vi "BK Precision 1696.vi"() -> ()   [LabVIEW 2020]
uses:
  SubVIs/BK_Precision1696_TypeDefinitions.llb/BK_1696_Output_On_OFF.ctl
  SubVIs/BK_Precision1696_TypeDefinitions.llb/BK_Precision1696_Steps.ctl
  LabVIEW 2020 Toolkits/toolkits_lv2020_32bit/Synchronization.llb/SynchRefs_SetGet.ctl
  LabVIEW 2020 Toolkits/VI Server Toolkit/VI Server Libraries/VI Server_Set Controls.llb/Set STR Control.vi
  LabVIEW 2020 Toolkits/VI Server Toolkit/VI Server Toolkit LV2013.lvlib
panel:
  out "InstrumentGood":bool caption="Instrument Good"
  out "InterfaceError":bool caption="Interface Error"
  out "CommandStatus":bool caption="Command Status"
  out "System.Message":string caption="System Message"
  in  "Help":bool
  in  "FP.Hide":bool caption="FrontPanel.Hide"
  in  "EXIT":bool
  in  "error in":errorcluster
  in  "Tab.Main":T1(tab)
  out "Indicator.CV":bool
  in  "Indicator.OVP.Set":dbl caption="Indicator.Current.Measured" format="%0.1f"
  in  "Indicator.Current.Set":dbl caption="Indicator.Current.Measured" format="%0.2f"
  in  "Indicator.Voltage.Set":dbl=0.1 caption="Indicator.Voltage.Measured" min=0.1 max=20.0 format="%0.1f "
  out "Indicator.Output.Enabled":T2
  in  "Indicator.Current.Measured":dbl format="%0.3f"
  in  "Indicator.Voltage.Measured":dbl format="%0.2f "
  in  "Indicator.Power.Measured":dbl format="%0.3f"
  in  "OVP.Level":dbl caption="OVP.Level.DUP" min=0.0 max=20.0 format="%0.1f V"
  in  "OVP.Level.DUP":dbl(knob) caption="Volts" min=0.0 max=20.0 scale=0.0..20.0
  in  "Output.Amps":dbl caption="Output.Amps.DUP" min=0.0 max=80.0 format="%0.3f A"
  in  "Output.Amps.DUP":dbl(knob) caption="Current Limit (Amp)" min=0.0 max=10.0 scale=0.0..10.0
  in  "Output.Volts":dbl=1.0 caption="Output.Volts.DUP" min=1.0 max=20.0 format="%0.1f V"
  in  "Output.Volts.DUP":dbl(knob)=1.0 caption="Volts" min=1.0 max=20.0 scale=1.0..20.0
  in  "Output.Enable":bool
  out "List.File.LoadedStep":string caption="Loaded Step"
  in  "List.File.#Cycles":u16 caption="# of Cycles" max=256 format="%03d"
  in  "List.File.Description":string caption="File Description"
  in  "List.File.Open":bool
  in  "List.File.RUN":bool
  in  "List.File.Load":bool
  in  "List.File.Save":bool
  in  "List.File":u16=1 caption="List File" min=1 max=100
  in  "Step.Parameters":T3 caption="Program Parameters" {"Seconds" max=59; "Minutes" max=99; "Step.Current" format="%0.2f A"; "Step.Voltage" format="%0.1f V"}
  in  "List.File.RUN.DUP":bool caption="List.File.RUN"
  out "Program.Progress":u8(slide) caption="Program Progress" scale=0.0..100.0
  out "Graph.TimeBetweenPoints":i32 caption="Time Between Points" format="%.0f msec"
  in  "Graph.Enable":bool
  out "Sequence.Graph":cluster{i32[], dbl[]}[](graph)
  in  "Instrument.Address":u8 caption="Instrument Address" max=31 format="%03d"
  in  "Measurements.AutoUpdate.Disable":bool
  in  "Measurements.UpdateRate":u32=100 caption="Measurements Update Rate" min=100 max=100000 format="%.0f msec"
  in  "VISA.Command2.Write":bool
  in  "VISA.Command2":string caption="Command"
  in  "VISA.Command.Write":bool
  in  "VISA.Command":string caption="Command"
  out "VISA.InstrumentResponce":string caption="Instrument Responce"
  in  "VISA.ResourceName":refnum<visa-resource-name>="BK_PRECISION_9115" caption="VISA Rresource Name"
  in  "UDP.Test.String2.Send":bool
  in  "UDP.Test.String2":string caption="UDP: Test String 2"
  in  "UDP.Port.Receiver":u16=58433 caption="UDP: Port.Receiver"
  in  "UDP.Port.Read":u16=58432 caption="UDP: Port.Read"
  in  "UDP.LocalPort.Write":u16=58434 caption="UDP: Local Port.Write"
  in  "UDP.IP.Address":string="234.5.6.7" caption="UDP: IP Address"
  in  "UDP.Test.String1.Send":bool
  in  "UDP.Test.String1":string caption="UDP: Test String 1"
  in  "UDP.Responce.String.Monitor":bool
  out "UDP.Responce.String":string caption="UDP: Responce String"
  in  "VI.WindowsTitle":string caption="Windows Title"
  out "error out":errorcluster={"status"=TRUE, "code"=1055, "source"="Property Node in VI Server Toolkit LV2013.lvlib:VI server_Set Control Value from String Format.vi:5200001->DMM6500_UDP_ExecEng_Instruction_APPLY.vi->DMM6500_UDP_MAIN.vi->Keithley2100.vi"}
  # "V"
  # "[SETTINGS]"
  # "V"
  # "V-set"
  # "A"
  # "A"
  # "W"
  # "V"
  # "OVP"
  # "OUTPUT"
  # "OUTPUT"
  # "OVERVOLTAGE"
  # "Step #               Voltage                  Current               Minute      Seconds"
  # "RS232 -> 000\nRS485 ->0 01 to 031"
  # "Multicast IP addresses must be in the 224.0.0.0 to 239.255.255.255 range."
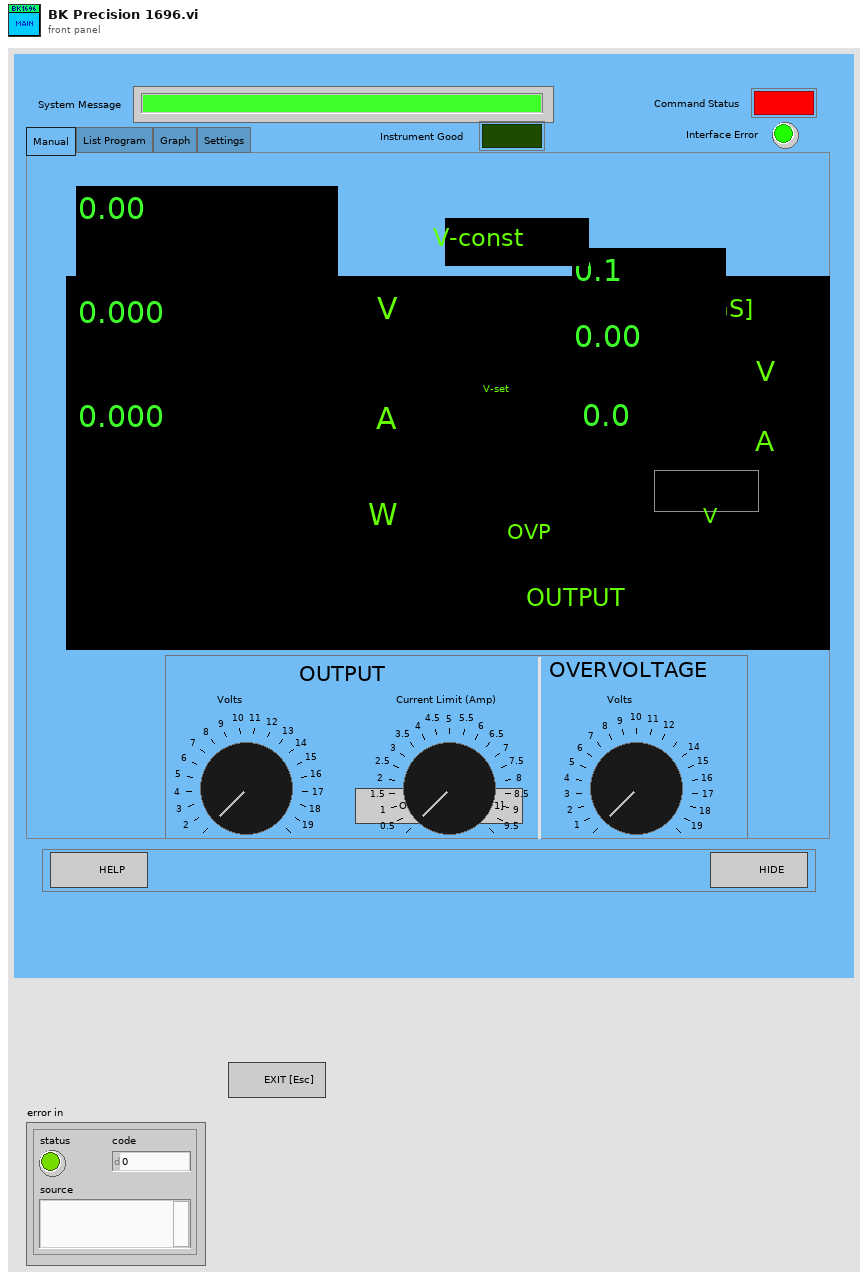
[diagram p1: front panel]
types:
  T1 = enum32{"Manual", "List Program", "Graph", "Settings"}
  T2 = typedef "BK_1696_Output_On_OFF.ctl" = bool
  T3 = typedef "BK_Precision1696_Steps.ctl" = cluster{"Step.Voltage":dbl, "Step.Current":dbl, "Minutes":u16, "Seconds":u16}[]
  T4 = typedef "VI Server_RefsCluster.ctl" = cluster{"Labels":string[], "Refs":refnum<vi>[], "VI Ref":refnum<vi>}
  T5 = typedef "SynchRefs_SetGet.ctl" = enum16{"Set", "Get"}
  T6 = cluster{"Step.Voltage":dbl, "Step.Current":dbl, "Step.Width":dbl, "Step.Slope":u8}[]
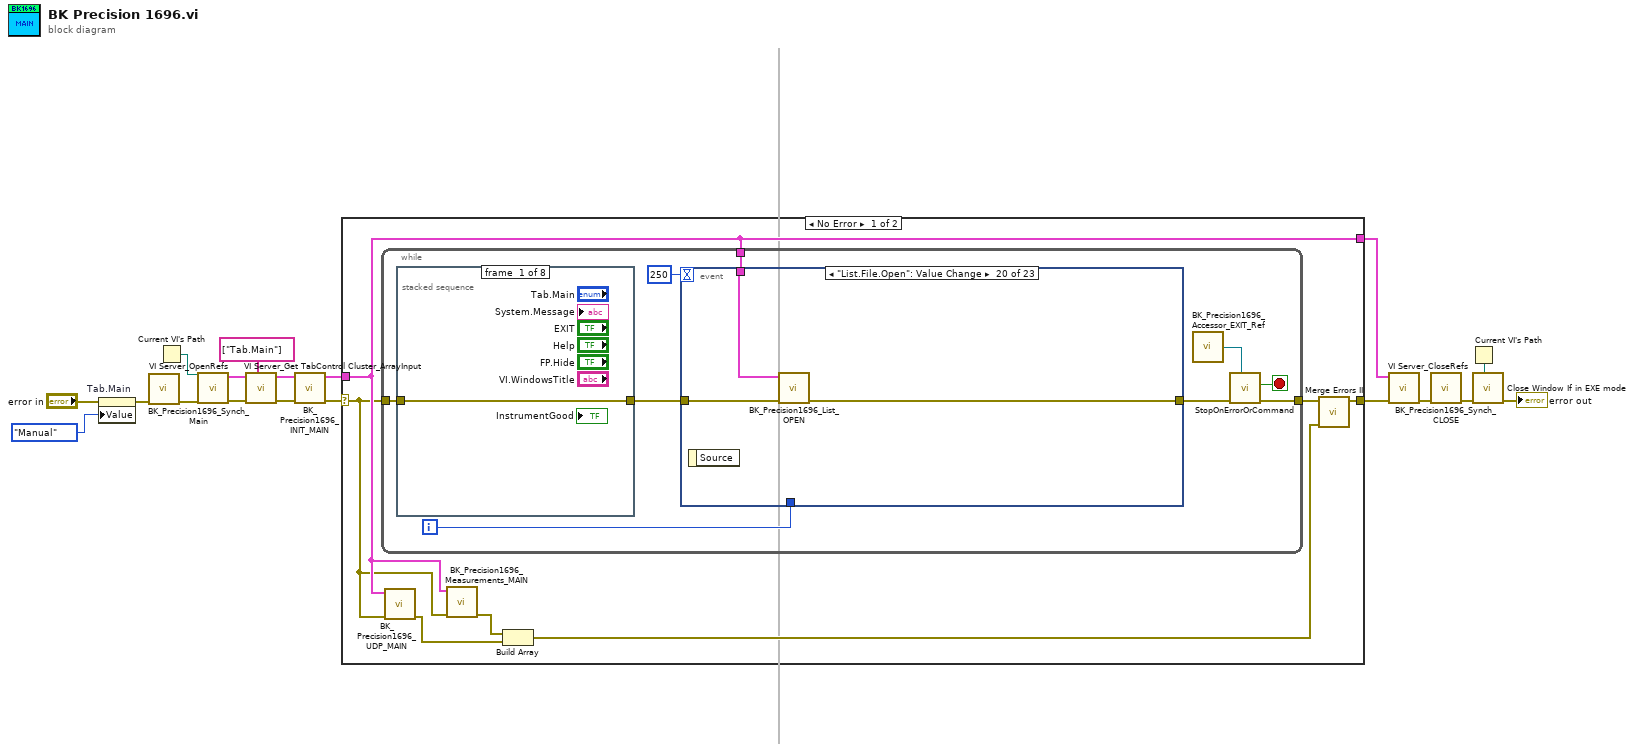
[diagram p0: block diagram]
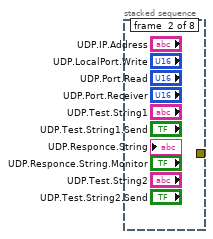
[diagram p2: hidden frame]
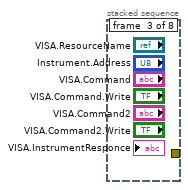
[diagram p3: hidden frame]
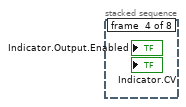
[diagram p4: hidden frame]
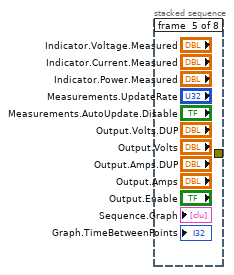
[diagram p5: hidden frame]
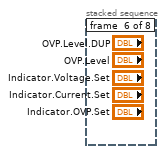
[diagram p6: hidden frame]
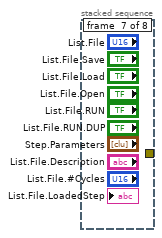
[diagram p7: hidden frame]
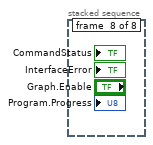
[diagram p8: hidden frame]
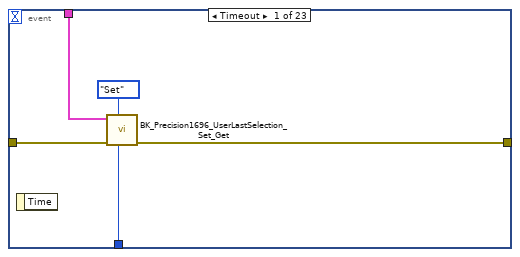
[diagram p9: hidden frame]
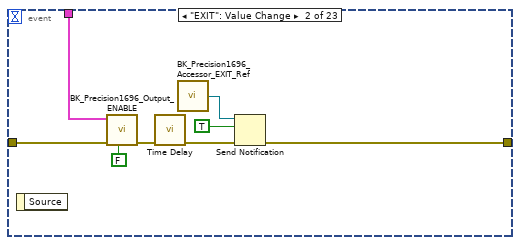
[diagram p10: hidden frame]
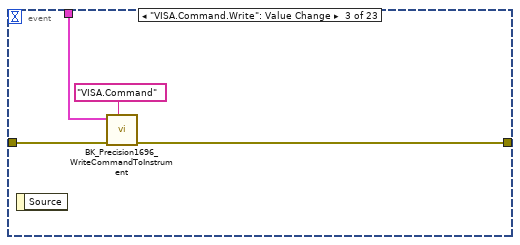
[diagram p11: hidden frame]
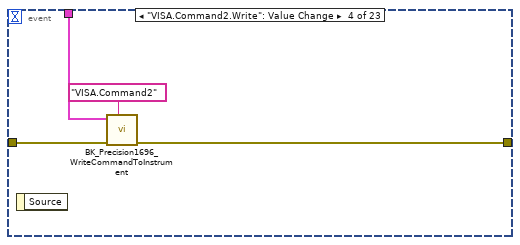
[diagram p12: hidden frame]
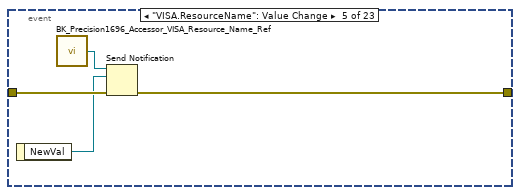
[diagram p13: hidden frame]
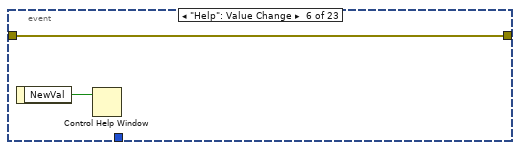
[diagram p14: hidden frame]
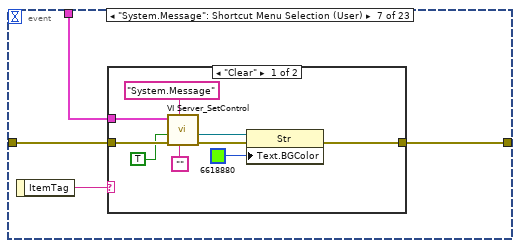
[diagram p15: hidden frame]
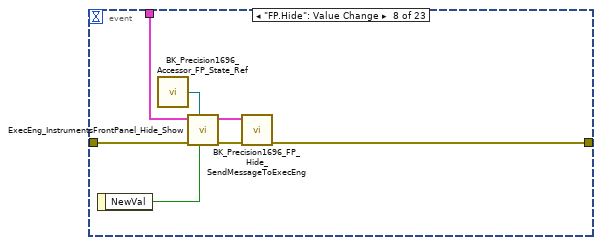
[diagram p17: hidden frame]
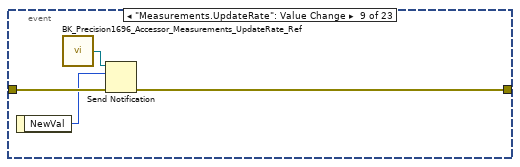
[diagram p18: hidden frame]
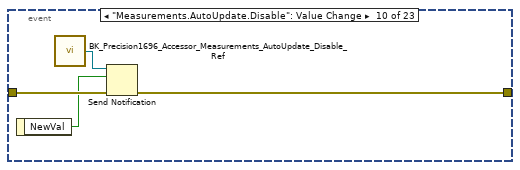
[diagram p19: hidden frame]
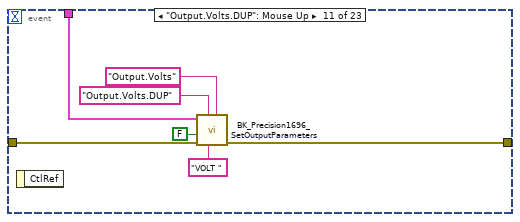
[diagram p20: hidden frame]
diagram:
  n1 = property on="Tab.Main" class="TabCtl (strict)"(error in="error in", "Value"=T1."Manual" ("Tab.Main")) -> (error out=w2:errorcluster)  [unwired: 1 in, 1 out]
  n2 = call "BK_Precision1696_Synch_Main.vi"("error in"=w2) -> ("error out"=w15:errorcluster)  [unwired: 10 in]
  n3 = Current VI's Path() -> (path=w17:path)
  n4 = call "VI Server_OpenRefs.vi"("error in"=w15, "VI Path"=w17) -> ("error out"=w14:errorcluster, "VI Server.RefsCluster"=w16:T4)  [unwired: 8 in]
  n5 = call "VI Server_Get TabControl Cluster_ArrayInput.vi"("TabControl Labels[]"=string[] ["Tab.Main"], "error in"=w14, "VI Server Cluster"=w16) -> ("error out"=w9:errorcluster, "VI Server Cluster.OUT"=w8:T4)  [unwired: 7 in]
  n6 = call "BK_Precision1696_INIT_MAIN.vi"("error in (no error)"=w9, "VI Server Cluster"=w8) -> ("error out"=w7:errorcluster, "VI Server Cluster DUP"=w5:T4)  [unwired: 8 in]
  n7 = case shown="No Error" w7 {
    selector: w7 -> [w22 w177]
    tunnel: [w24 w177] -> w6
    tunnel: w5 -> [w23 w176]
    tunnel: [w23 w176] -> w4
    frame No Error {
      n8 = while {
        tunnel: w22 -> [w34]
        tunnel: w23 -> [w31]
        tunnel: [w27] -> w25
        i -> [w30]
        stop <- w26 stop-if-true
        n9 = stacked-sequence {
          tunnel: w34 -> [w35 _ _ _ _ _ _ _]
          tunnel: [w35 _ _ _ _ _ _ _] -> w32
          frame #0 {
          }
          frame #1 {
          }
          frame #2 {
          }
          frame #3 {
          }
          frame #4 {
          }
          frame #5 {
          }
          frame #6 {
          }
          frame #7 {
          }
        }
        n10 = event shown="[19] \"List.File.Open\": Value Change" {
          selector: _ -> [_ _ _ _ _ _ _ _ _ _ _ _ _ _ _ _ _ _ _ _ _ _ _]
          dyn-events: _ -> [_ _ _ _ _ _ _ _ _ _ _ _ _ _ _ _ _ _ _ _ _ _ _]
          timeout: 250 -> [_ _ _ _ _ _ _ _ _ _ _ _ _ _ _ _ _ _ _ _ _ _ _]
          tunnel: w32 -> [w40 w44 w52 w56 w60 w61 w65 w83 w87 w91 w97 w104 w111 w118 w122 w129 w136 w151 w160 w163 w166 w171 w175]
          tunnel: w31 -> [w39 w45 w51 w55 _ _ w63 w81 _ _ w96 w103 w110 w117 w121 w128 w135 w152 w159 w162 w164 w170 _]
          tunnel: [w36 w47 w50 w54 w57 w61 w64 w78 w84 w89 w98 w105 w112 w119 w123 w130 w137 w142 w158 w161 w165 w169 w172] -> w28
          tunnel: w30 -> [w38 _ _ _ _ _ _ _ _ _ _ _ _ _ _ _ _ _ _ _ _ _ _]
          event Timeout {
            n11 = event-data() -> ()  [unwired: 1 in, 1 out]
            n12 = call "BK_Precision1696_UserLastSelection_Set_Get.vi"("LoopCounter"=w38, "SynchRefs.Set/Get"=SynchRefs_SetGet."Set", "error in"=w40, "VI Server.RefsCluster"=w39) -> ("error out"=w36:errorcluster)  [unwired: 6 in, 1 out]
          }
          event "EXIT": Value Change {
            n13 = event-data() -> ()  [unwired: 1 in, 1 out]
            n14 = call "BK_Precision1696_Output_ENABLE.vi"("Output.Enable"=FALSE, "error in (no error)"=w44, "VI Server Cluster"=w45) -> ("error out"=w41:errorcluster)  [unwired: 8 in]
            n15 = call "Time Delay"("error in (no error)"=w41) -> ("error out"=w42:errorcluster)  [unwired: 10 in]
            n16 = call "BK_Precision1696_Accessor_EXIT_Ref.vi"() -> ("EXIT"=w48:refnum<notifier>)  [unwired: 6 in]
            n17 = Send Notification(notification=TRUE, notifier=w48, error in (no error)=w42) -> (error out=w47:errorcluster)  [unwired: 1 out]
          }
          event "VISA.Command.Write": Value Change {
            n18 = event-data() -> ()  [unwired: 1 in, 1 out]
            n19 = call "BK_Precision1696_WriteCommandToInstrument.vi"("Control.Label"="VISA.Command", "error in (no error)"=w52, "VI Server Cluster"=w51) -> ("error out"=w50:errorcluster)  [unwired: 8 in]
          }
          event "VISA.Command2.Write": Value Change {
            n20 = event-data() -> ()  [unwired: 1 in, 1 out]
            n21 = call "BK_Precision1696_WriteCommandToInstrument.vi"("Control.Label"="VISA.Command2", "error in (no error)"=w56, "VI Server Cluster"=w55) -> ("error out"=w54:errorcluster)  [unwired: 8 in]
          }
          event "VISA.ResourceName": Value Change {
            n22 = event-data() -> ("NewVal"=w58:refnum<visa-resource-name>)  [unwired: 1 in]
            n23 = call "BK_Precision1696_Accessor_VISA_Resource_Name_Ref.vi"() -> ("VISA resource name"=w59:refnum<notifier>)  [unwired: 6 in]
            n24 = Send Notification(notification=w58, notifier=w59, error in (no error)=w60) -> (error out=w57:errorcluster)  [unwired: 1 out]
          }
          event "Help": Value Change {
            n25 = event-data() -> ("NewVal"=w62:bool)  [unwired: 1 in]
            n26 = Control Help Window(1:w62) -> ()  [unwired: 1 in]
          }
          event "System.Message": Shortcut Menu Selection (User) {
            n27 = event-data() -> ("ItemTag"=w66:string)  [unwired: 1 in]
            n28 = case shown="\"Clear\"" w66 {
              tunnel: w65 -> [w71 w76]
              tunnel: [w72 w76] -> w64
              tunnel: w63 -> [w69 _]
              frame "Clear" {
                n29 = call-poly "VI Server_SetControl.vi"("New Value"="", "Label"="System.Message", "error in"=w71, "Single Instance (T)"=TRUE ("SingleInstance"), "VI Server Cluster"=w69) -> ("error out"=w74:errorcluster, "Control Ref"=w75:refnum<vi>)  [unwired: 4 in, 1 out]
                n30 = property class="Str"(reference=w75, error in=w74, "Text.BGColor"=u32 6618880) -> (error out=w72:errorcluster)  [unwired: 1 out]
              }
              frame "", Default {
              }
            }
          }
          event "FP.Hide": Value Change {
            n31 = event-data() -> ("NewVal"=w82:bool)  [unwired: 1 in]
            n32 = call "BK_Precision1696_Accessor_FP_State_Ref.vi"() -> ("FP.State"=w80:refnum<notifier>)  [unwired: 6 in]
            n33 = call "ExecEng_InstrumentsFrontPanel_Hide_Show.vi"("FP.Hide/Show"=w82, "FP.State"=w80, "error in (no error)"=w83, "VI Server Cluster"=w81) -> ("error out"=w79:errorcluster, "VI Server Cluster DUP"=w77:T4)  [unwired: 6 in]
            n34 = call "BK_Precision1696_FP_Hide_SendMessageToExecEng.vi"("error in (no error)"=w79, "VI Server Cluster"=w77) -> ("error out"=w78:errorcluster)  [unwired: 9 in]
          }
          event "Measurements.UpdateRate": Value Change {
            n35 = event-data() -> ("NewVal"=w85:u32)  [unwired: 1 in]
            n36 = call "BK_Precision1696_Accessor_Measurements_UpdateRate_Ref.vi"() -> ("Measurements.UpdateRate"=w86:refnum<notifier>)  [unwired: 6 in]
            n37 = Send Notification(notification=w85, notifier=w86, error in (no error)=w87) -> (error out=w84:errorcluster)  [unwired: 1 out]
          }
          event "Measurements.AutoUpdate.Disable": Value Change {
            n38 = event-data() -> ("NewVal"=w90:bool)  [unwired: 1 in]
            n39 = call "BK_Precision1696_Accessor_Measurements_AutoUpdate_Disable_Ref.vi"() -> ("Measurements.AutoUpdate.Disable"=w88:refnum<notifier>)  [unwired: 6 in]
            n40 = Send Notification(notification=w90, notifier=w88, error in (no error)=w91) -> (error out=w89:errorcluster)  [unwired: 1 out]
          }
          event "Output.Volts.DUP": Mouse Up {
            n41 = event-data() -> ()  [unwired: 1 in, 1 out]
            n42 = call "BK_Precision1696_SetOutputParameters.vi"("DuplicateControl.Label"="Output.Volts" ("Control.Label"), "Command.Template"="VOLT " ("Set Voltage"), "Control.Label"="Output.Volts.DUP", "error in (no error)"=w97, "DisableSemaphor"=FALSE, "VI Server Cluster"=w96) -> ("error out"=w98:errorcluster)  [unwired: 4 in, 1 out]
          }
          event "Output.Volts": Value Change {
            n43 = event-data() -> ()  [unwired: 1 in, 1 out]
            n44 = call "BK_Precision1696_SetOutputParameters.vi"("DuplicateControl.Label"="Output.Volts.DUP" ("Control.Label"), "Command.Template"="VOLT" ("Set Voltage"), "Control.Label"="Output.Volts", "error in (no error)"=w104, "DisableSemaphor"=FALSE, "VI Server Cluster"=w103) -> ("error out"=w105:errorcluster)  [unwired: 4 in, 1 out]
          }
          event "Output.Amps.DUP": Mouse Up {
            n45 = event-data() -> ()  [unwired: 1 in, 1 out]
            n46 = call "BK_Precision1696_SetOutputParameters.vi"("DuplicateControl.Label"="Output.Amps" ("Control.Label"), "Command.Template"="CURR" ("Set Voltage"), "Control.Label"="Output.Amps.DUP", "error in (no error)"=w111, "DisableSemaphor"=FALSE, "VI Server Cluster"=w110) -> ("error out"=w112:errorcluster)  [unwired: 4 in, 1 out]
          }
          event "Output.Amps": Value Change {
            n47 = event-data() -> ()  [unwired: 1 in, 3 out]
            n48 = call "BK_Precision1696_SetOutputParameters.vi"("DuplicateControl.Label"="Output.Amps.DUP" ("Control.Label"), "Command.Template"="CURR" ("Set Voltage"), "Control.Label"="Output.Amps", "error in (no error)"=w118, "DisableSemaphor"=FALSE, "VI Server Cluster"=w117) -> ("error out"=w119:errorcluster)  [unwired: 4 in, 1 out]
          }
          event "Output.Enable": Value Change {
            n49 = event-data() -> ("NewVal"=w120:bool)  [unwired: 1 in]
            n50 = call "BK_Precision1696_Output_ENABLE.vi"("Output.Enable"=w120, "error in (no error)"=w122, "VI Server Cluster"=w121) -> ("error out"=w123:errorcluster)  [unwired: 8 in]
          }
          event "OVP.Level.DUP": Mouse Up {
            n51 = event-data() -> ()  [unwired: 1 in, 1 out]
            n52 = call "BK_Precision1696_SetOutputParameters.vi"("DuplicateControl.Label"="OVP.Level" ("Control.Label"), "Command.Template"="SOVP" ("Set Voltage"), "Control.Label"="OVP.Level.DUP", "error in (no error)"=w129, "DisableSemaphor"=FALSE, "VI Server Cluster"=w128) -> ("error out"=w130:errorcluster)  [unwired: 4 in, 1 out]
          }
          event "OVP.Level": Value Change {
            n53 = event-data() -> ()  [unwired: 1 in, 1 out]
            n54 = call "BK_Precision1696_SetOutputParameters.vi"("DuplicateControl.Label"="OVP.Level.DUP" ("Control.Label"), "Command.Template"="SOVP" ("Set Voltage"), "Control.Label"="OVP.Level", "error in (no error)"=w136, "DisableSemaphor"=FALSE, "VI Server Cluster"=w135) -> ("error out"=w137:errorcluster)  [unwired: 4 in, 1 out]
          }
          event Mouse Up {
            n55 = event-data() -> ()  [unwired: 1 in, 1 out]
            n56 = call "BK_Precision1696_ProgramSteps_Set_Get.vi"("Value.In"=T6 [], "SynchRefs.Set/Get"=SynchRefs_SetGet."Get", "error in (no error)"=w151, "VI Server Cluster"=w152) -> ("error out"=w149:errorcluster, "Ref"=w147:refnum<vi>)  [unwired: 4 in, 2 out]
            n57 = property class="Arr (strict)"(reference=w147, error in=w149) -> (reference out=w141:refnum<vi>, error out=w143:errorcluster, "Index Values"=w146:u32[])
            n58 = Index Array(array=w146) -> (element=w145:u32)  [unwired: 1 in]
            n59 = Greater?(x=w145, y=u32 20) -> (0:w138:bool)
            n60 = Build Array(u32 20 ("y")) -> (w139:u32[])
            n61 = case shown="True" w138 {
              tunnel: w143 -> [w153 w157]
              tunnel: [w153 w156] -> w142
              tunnel: w141 -> [_ w155]
              tunnel: w139 -> [_ w154]
              frame False {
              }
              frame True {
                n62 = property class="Arr (strict)"(reference=w155, error in=w157, "Index Values"=w154) -> (error out=w156:errorcluster)  [unwired: 1 out]
              }
            }
          }
          event "List.File.Save": Value Change {
            n63 = event-data() -> ()  [unwired: 1 in, 1 out]
            n64 = call "BK_Precision1696_List_SAVE.vi"("error in (no error)"=w160, "VI Server Cluster"=w159) -> ("error out"=w158:errorcluster)  [unwired: 9 in]
          }
          event "List.File.Open": Value Change {
            n65 = event-data() -> ()  [unwired: 1 in, 1 out]
            n66 = call "BK_Precision1696_List_OPEN.vi"("error in (no error)"=w163, "VI Server Cluster"=w162) -> ("error out"=w161:errorcluster)  [unwired: 9 in]
          }
          event "List.File.Load": Value Change {
            n67 = event-data() -> ()  [unwired: 1 in, 1 out]
            n68 = call "BK_Precision1696_List_LOAD.vi"("error in (no error)"=w166, "VI Server Cluster"=w164) -> ("error out"=w165:errorcluster)  [unwired: 9 in]
          }
          event "List.File.RUN", "List.File.RUN.DUP": Value Change {
            n69 = event-data() -> ("NewVal"=w168:bool, "CtlRef"=w167:refnum<vi>)  [unwired: 1 in]
            n70 = call "BK_Precision1696_List_RUN.vi"("CtlRef"=w167, "List.File.RUN"=w168, "error in (no error)"=w171, "VI Server Cluster"=w170) -> ("error out"=w169:errorcluster)  [unwired: 7 in]
          }
          event "Graph.Enable": Value Change {
            n71 = event-data() -> ("NewVal"=w173:bool)  [unwired: 1 in]
            n72 = call "BK_Precision1696_Accessor_Graph_Enable_Ref.vi"() -> ("Graph.Enable"=w174:refnum<notifier>)  [unwired: 6 in]
            n73 = Send Notification(notification=w173, notifier=w174, error in (no error)=w175) -> (error out=w172:errorcluster)  [unwired: 1 out]
          }
        }
        n74 = call "BK_Precision1696_Accessor_EXIT_Ref.vi"() -> ("EXIT"=w29:refnum<notifier>)  [unwired: 6 in]
        n75 = call "StopOnErrorOrCommand.vi"("STOP"=w29, "error in (no error)"=w28) -> ("error out"=w27:errorcluster, "STOP"=w26:bool)  [unwired: 8 in]
      }
      n76 = call "BK_Precision1696_UDP_MAIN.vi"("error in (no error)"=w22, "VI Server.RefsCluster"=w23) -> ("error out"=w20:errorcluster)  [unwired: 9 in]
      n77 = call "BK_Precision1696_Measurements_MAIN.vi"("error in (no error)"=w22, "VI Server.RefsCluster"=w23) -> ("error out"=w21:errorcluster)  [unwired: 9 in]
      n78 = Build Array(w21, w20) -> (w19:errorcluster[])
      n79 = call "Merge Errors II.vi"("error array in"=w19, "error in 1 (no error)"=w25) -> ("error out.DUP"=w24:errorcluster)  [unwired: 4 in, 1 out]
    }
    frame Error {
    }
  }
  n80 = call "VI Server_CloseRefs.vi"("error in"=w6, "VI Server.RefsCluster"=w4) -> ("error out"=w12:errorcluster)  [unwired: 9 in]
  n81 = call "BK_Precision1696_Synch_CLOSE.vi"("error in"=w12) -> ("error out"=w11:errorcluster)  [unwired: 10 in]
  n82 = Current VI's Path() -> (path=w18:path)
  n83 = call "Close Window If in EXE mode.vi"("TopLevelVI Path"=w18, "error in"=w11) -> ("error out"=→"error out":errorcluster)  [unwired: 9 in]
